vi "Common_UpdateAttributes.vi"(1 "ClassPath/LvClassRef":variant, 2 "NewAttributes":string, 3 "ClassInfo":T4[](array[typedef]), 5 "error in (no error)":errorcluster, 6 "Don't Prompt (False)":bool, 7 "Attributes":T1[](array[typedef]), 8 "Stereotype":string, 9 "Ctl-Description":string) -> (15 "CtlPath":path, 18 "Cancel":bool, 19 "error out":errorcluster)   [LabVIEW 2020] (continued)
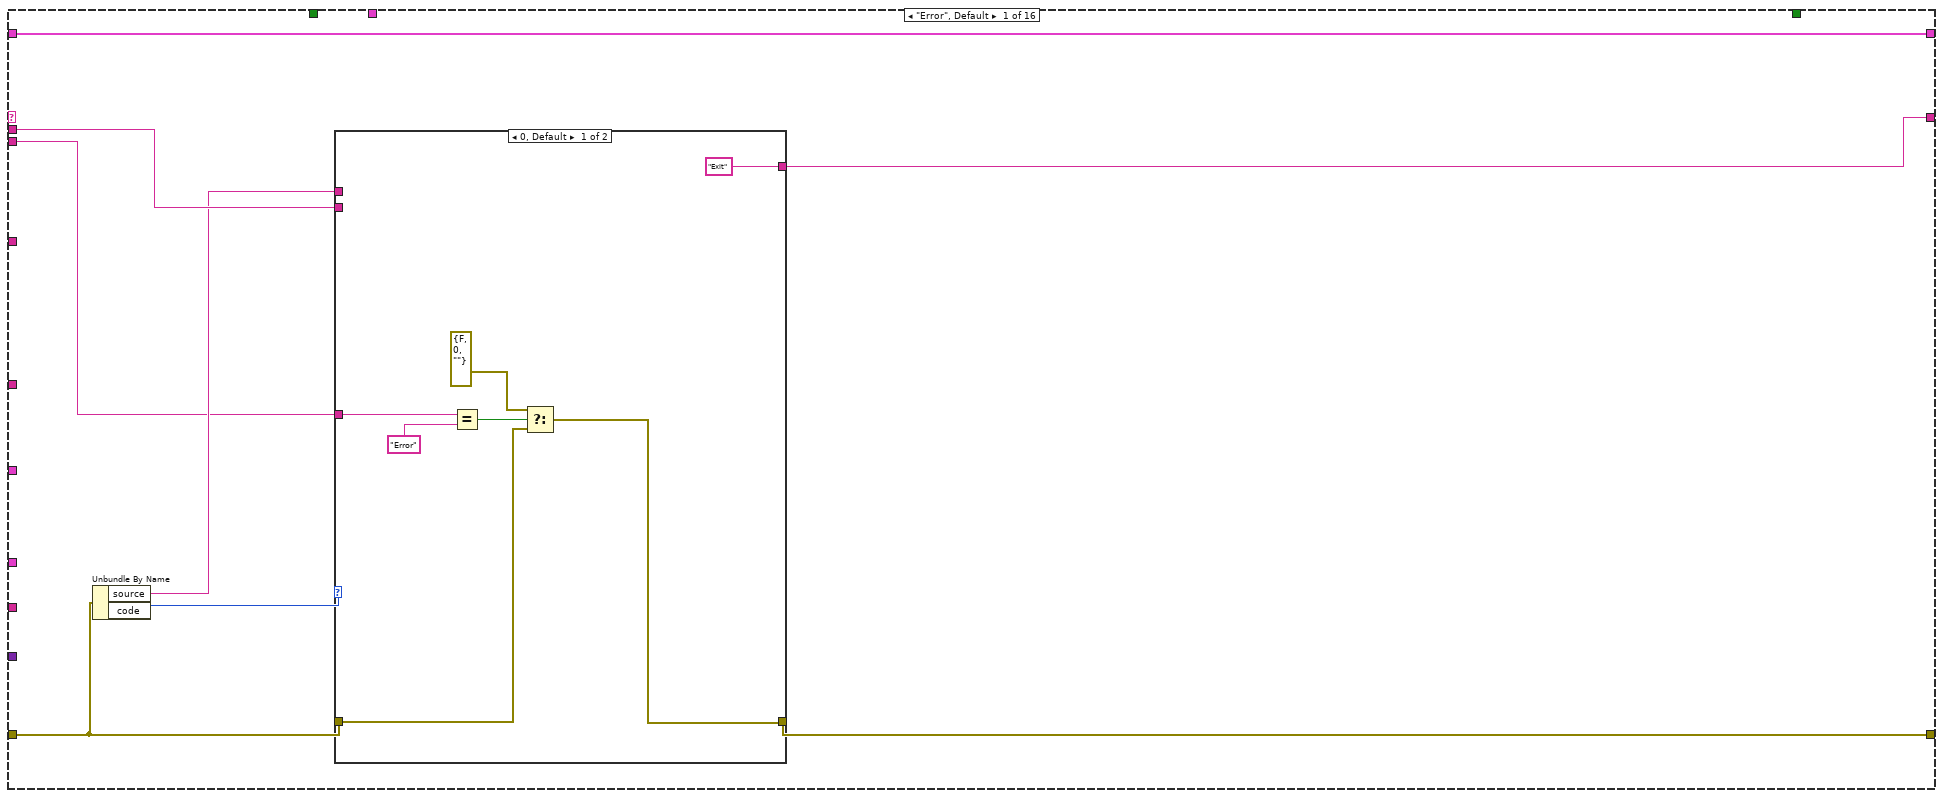
[diagram p3: hidden frame]
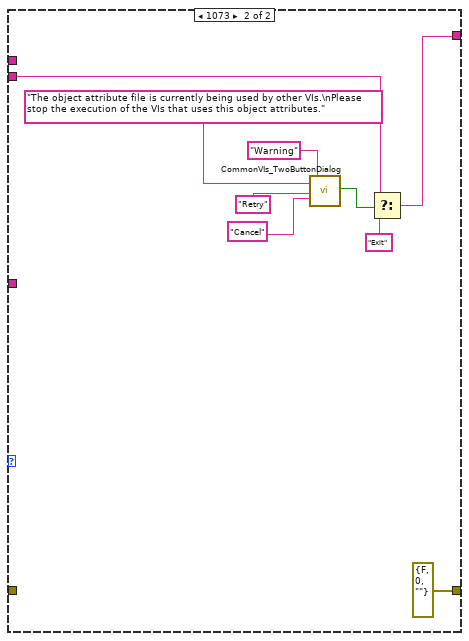
[diagram p4: hidden frame]
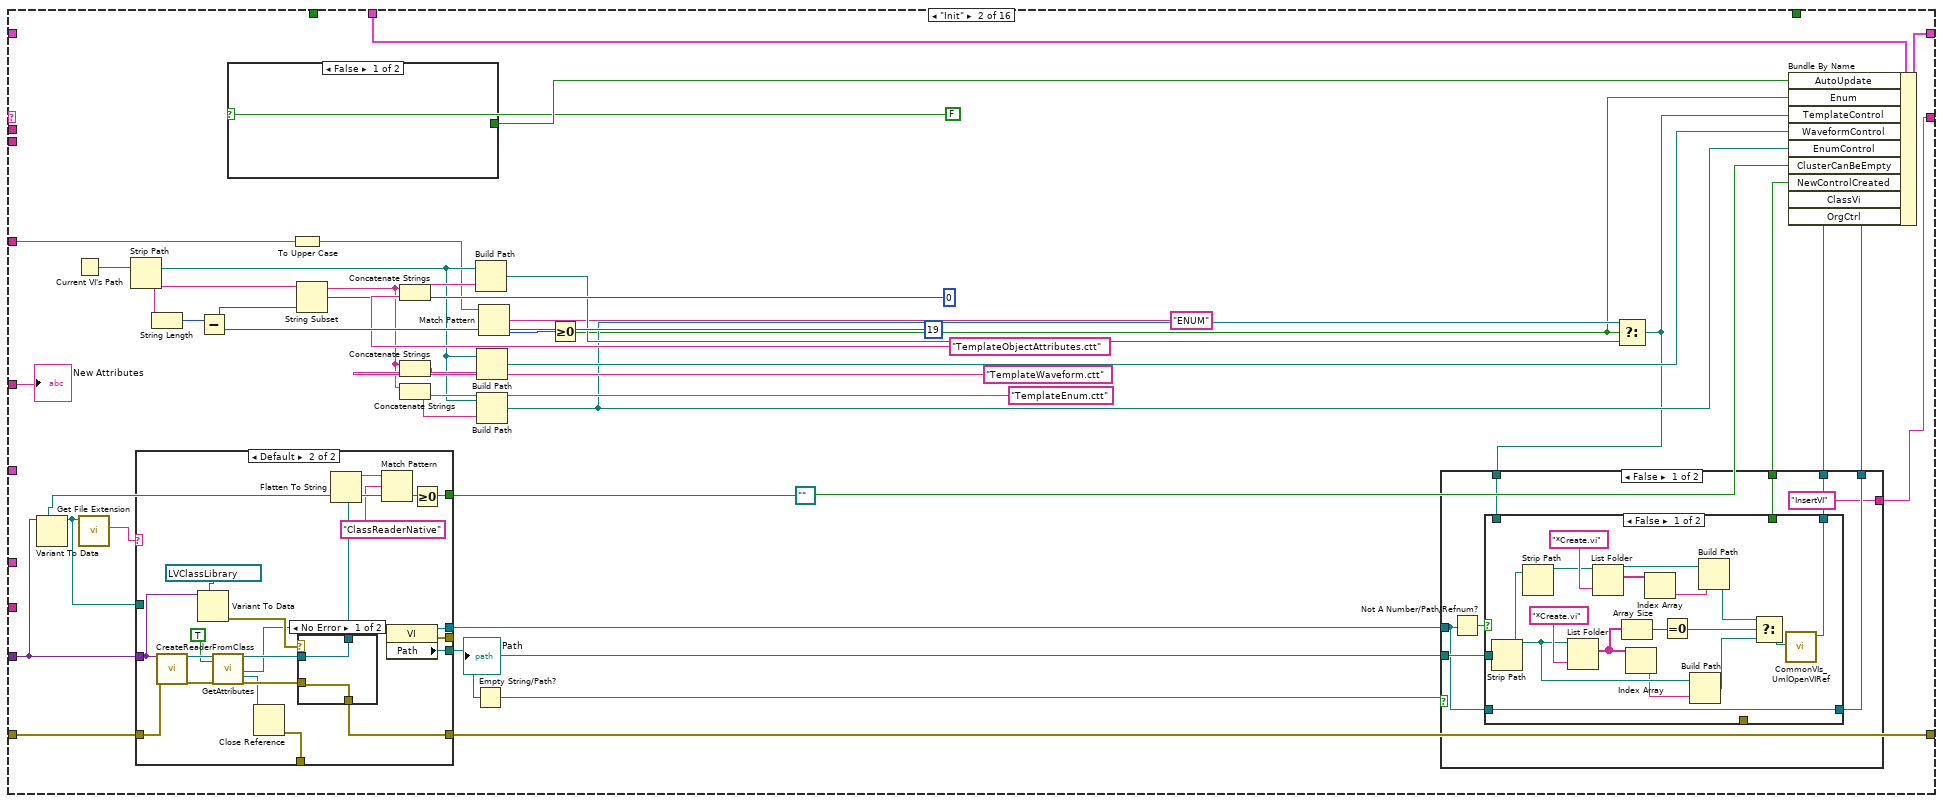
[diagram p5: hidden frame]
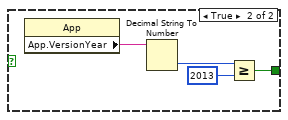
[diagram p6: hidden frame]
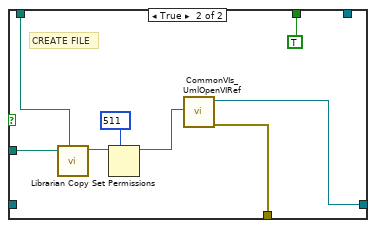
[diagram p7: hidden frame]
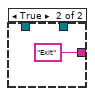
[diagram p8: hidden frame]
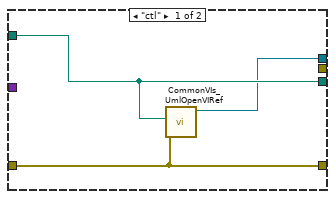
[diagram p9: hidden frame]
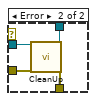
[diagram p10: hidden frame]
                  n285 = Close Reference(reference=w814, error in (no error)=w826) -> (error out=w832:errorcluster)
                  n286 = for {
                    tunnel: w806 -> [w838] mode=indexing
                    tunnel: w799 -> [_]
                    n287 = Close Reference(reference=w838) -> ()  [unwired: 1 in, 1 out]
                  }
                  n288 = invoke on="EmptyClip" class="App" method="Clipboard.Empty"(error in=w832) -> (error out=w833:errorcluster)  [unwired: 2 in, 2 out]
                }
              }
              n289 = property class="Ctl"(reference=w535, error in=w544, "Label.Text"=w515, "Auto-Update From Typedef"=TRUE ("Label.Visible")) -> (reference out=w540:refnum<vi>, error out=w545:errorcluster)
              n290 = property class="Ctl"(reference=w540, error in=w545, "Label.Text"=w515, "Label.Visible"=TRUE) -> (reference out=w541:refnum<vi>, error out=w543:errorcluster)
            }
            n291 = Array Size(array=w487) -> (size(s)=w484:i32)
            n292 = Equal?(x=w485, y=w484) -> (x = y?=w483:bool)
            n293 = And Array Elements(Boolean array=w487) -> (logical AND=w488:bool)
            n294 = And(x=w483, y=w488) -> (x .and. y?=w482:bool)
            n295 = Build Array (concatenate)(w502, w500) -> (w501:refnum<vi>[])
            n296 = Bundle By Name(cluster=w491, "NoUpdate"=w482, "AddedCtrls"=w501) -> (w503:T5)
          }
          frame "Move Controls" {
            n297 = Unbundle By Name(w845) -> ("NewCtrl"=w856:refnum<vi>, "NewCluster"=w855:refnum<vi>, "OrgCtrl"=w852:refnum<vi>, "OrgCluster"=w853:refnum<vi>, "NewEnum"=w846:refnum<vi>)
            n298 = property class="VI"(reference=w852) -> ("Front Panel Window:Origin"=w854:T13)  [unwired: 1 in, 2 out]
            n299 = property class="VI"(reference=w856) -> ("Front Panel Window:Origin"=w847:T13)  [unwired: 1 in, 2 out]
            n300 = property class="Clust"(reference=w853, "Position"=w854) -> ()  [unwired: 1 in, 2 out]
            n301 = property class="Clust"(reference=w855, "Position"=w847) -> ()  [unwired: 1 in, 2 out]
            n302 = property class="Enum"(reference=w846, "Position"=w847) -> ()  [unwired: 1 in, 2 out]
            n303 = case shown="True" FALSE {
              tunnel: [_ w858] -> w841
              frame False {
              }
              frame True {
                n304 = property class="App"() -> ("App.VersionYear"=w861:string)  [unwired: 2 in, 2 out]
                n305 = Decimal String To Number(string=w861) -> (number=w860:i32)  [unwired: 2 in, 1 out]
                n306 = Greater Or Equal?(x=w860, y=2013) -> (x >= y?=w858:bool)
              }
            }
            n307 = Unbundle By Name(w845) -> ("NoUpdate"=w843:bool, "AutoUpdate"=w842:bool, "NewControlCreated"=w839:bool)
            n308 = Compound Arithmetic op=OR(w848, w843, w842, w839, w841) -> (w844:bool)
            n309 = Select(t="SaveCtrl" ("y"), s=w844, f="Idle" ("y")) -> (s? t:f=w849:string)
          }
          frame "Idle" {
            n310 = Unbundle By Name(w870) -> ("NewCluster"=w869:refnum<vi>, "OrgCtrl"=w862:refnum<vi>)  [unwired: 1 out]
            n311 = while {
              tunnel: [w881] -> w871
              tunnel: w862 -> [w880]
              stop <- w879 stop-if-true
              n312 = event shown="[3] Panel Close?" {
                selector: _ -> [_ _ _ _]
                dyn-events: _ -> [_ _ _ _]
                timeout: 500 -> [_ _ _ _]
                tunnel: ["Cancel" _ _ TRUE ("Cancel")] -> w881
                tunnel: w880 -> [_ w895 _ _]
                tunnel: [TRUE _ _ TRUE] -> w879
                event "OK", "Cancel": Value Change {
                  n313 = event-data() -> ()  [unwired: 2 out]
                  n314 = case shown="True" "OK" {
                    frame False {
                    }
                    frame True {
                      n315 = call <vilib>:"Set Busy.vi"() -> ()  [unwired: 4 in, 8 out]
                    }
                  }
                }
                event "Backup": Value Change {
                  n316 = event-data() -> ()  [unwired: 2 out]
                  n317 = call <vilib>:"Dflt Data Dir.vi"() -> ("App:Default Data Directory"=w905:path)
                  n318 = Format Date/Time String(time format string (%c)="%y%m%d_%H%M%S_") -> (date/time string=w900:string)  [unwired: 2 out]
                  n319 = property class="VI"(reference=w895) -> (reference out=w896:refnum<vi>, error out=w906:errorcluster, "VI Name"=w887:string)  [unwired: 1 in]
                  n320 = Build Path(base path=w905, name or relative path="Backup") -> (appended path=w901:path)
                  n321 = Match Pattern(string=w887, regular expression=":") -> (after substring=w886:string)  [unwired: 4 out]
                  n322 = Create Folder(path (use dialog)=w901) -> (created path=w890:path)  [unwired: 1 in, 3 out]
                  n323 = Concatenate Strings(w900, w886) -> (w891:string)
                  n324 = Build Path(base path=w890, name or relative path=w891) -> (appended path=w893:path)
                  n325 = Format Into String(format string="Do you want to save a backup file\nof the original control here.\n\n%s", w893) -> (resulting string=w902:string)  [unwired: 2 in, 1 out]
                  n326 = Two Button Dialog(message=w902, 1:"No" ("F button name (\"Cancel\")"), 2:"Yes" ("T button name (\"OK\")")) -> (T button?=w894:bool)
                  n327 = case shown="False" w894 {
                    tunnel: w893 -> [_ w914]
                    tunnel: [w910 w914] -> w892
                    tunnel: w891 -> [w912 _]
                    tunnel: w890 -> [w911 _]
                    tunnel: [w909 _] -> w889
                    tunnel: "Select backup file path" ("prompt") -> [w908 _]
                    frame False {
                      (unwired) T14."new or existing file" ("select mode (2)")
                      n328 = File Dialog(5:"Save" ("button label"), 6:"*.ctl" ("default name"), 7:w908, 9:w912, 11:w911) -> (1:w909:bool, 3:w910:path)  [unwired: 1 in, 3 out]
                    }
                    frame True {
                    }
                  }
                  n329 = case shown="False" w889 {
                    tunnel: w906 -> [w920 w922]
                    tunnel: w896 -> [w916 w921]
                    tunnel: w892 -> [w918 _]
                    tunnel: [w917 w921] -> _
                    tunnel: [w919 w922] -> _
                    frame False {
                      n330 = invoke class="VI" method="Save.Instrument"(reference=w916, error in=w920, "Path to saved file"=w918, "Save a Copy"=TRUE) -> (reference out=w917:refnum<vi>, error out=w919:errorcluster)  [unwired: 2 in, 4 out]
                    }
                    frame True {
                    }
                  }
                }
                event Timeout {
                  n331 = event-data() -> ()  [unwired: 2 out]
                  n332 = property class="VI"("Front Panel Window:Is Frontmost"=TRUE) -> ()  [unwired: 2 in, 2 out]
                }
                event Panel Close? {
                  n333 = event-data() -> ()  [unwired: 2 out]
                  n334 = event-data("Discard?"=TRUE) -> ()  [unwired: 1 in, 1 out]
                }
              }
            }
            n335 = property class="Clust"(reference=w869, "Auto Sizing"=u32 3) -> ("Controls[]"=w863:refnum<vi>[])  [unwired: 1 in, 2 out]
            n336 = Index Array(array=w863) -> (element=w867:refnum<vi>)  [unwired: 1 in]
            n337 = property class="Ctl"(reference=w867) -> (reference out=w866:refnum<vi>, "Position:Left"=w865:i32)  [unwired: 1 in, 1 out]
            n338 = Increment(x=w865) -> (x+1=w864:i32)
            n339 = property class="Ctl"(reference=w866, "Position:Left"=w864) -> (error out=w876:errorcluster)  [unwired: 1 in, 1 out]
            n340 = for {
              tunnel: w863 -> [w927] mode=indexing
              tunnel: w876 -> [_]
              n341 = Close Reference(reference=w927) -> ()  [unwired: 1 in, 1 out]
            }
            n342 = invoke class="VI" method="FP.Open"() -> ()  [unwired: 5 in, 5 out]
            n343 = Bundle By Name(cluster=w870, "Cancel"=w871) -> (w872:T5)
            n344 = Select(t="Exit" ("y"), s=w871, f="SaveCtrl" ("y")) -> (s? t:f=w873:string)
          }
          frame "SaveCtrl" {
            n345 = Unbundle By Name(w935) -> ("NewEnum"=w929:refnum<vi>, "OrgCluster"=w933:refnum<vi>, "OrgCtrl"=w928:refnum<vi>)  [unwired: 1 out]
            n346 = stacked-sequence {
              tunnel: w940 -> [w945]
              tunnel: [w945] -> w936
              tunnel: [w944] -> _
              tunnel: [w943] -> _
              frame #0 {
                n347 = invoke on="Attribute Before" class="SubPanel" method="Remove VI"() -> (error out=w944:errorcluster)  [unwired: 3 in, 2 out]
                n348 = invoke on="Attribute After" class="SubPnl" method="Remove VI"() -> (error out=w943:errorcluster)  [unwired: 3 in, 2 out]
              }
            }
            n349 = property class="VI"(reference=w928, error in=w936, "Front Panel Window:Origin"=cluster{"Horizontal":i16, "Vertical":i16} {"Horizontal"=0, "Vertical"=0}) -> (error out=w937:errorcluster)  [unwired: 1 out]
            n350 = property class="Clust"(reference=w933, error in=w937, "Position"=cluster{"Left":i32, "Top":i32} {"Left"=5, "Top"=5}) -> (error out=w938:errorcluster)  [unwired: 1 out]
            n351 = property class="Enum"(reference=w929, error in=w937, "Position"=cluster{"Left":i32, "Top":i32} {"Left"=5, "Top"=5}) -> (error out=w939:errorcluster)  [unwired: 1 out]
            n352 = stacked-sequence {
              tunnel: w937 -> [w941]
              tunnel: w939 -> [_]
              tunnel: w938 -> [_]
              frame #0 {
                n353 = disable-structure shown="Disabled" {
                  disable-tunnel: w941 -> [w942 _]
                  frame Disabled {
                    n354 = invoke class="VI" method="Save.Instrument"(error in=w942) -> ()  [unwired: 5 in, 6 out]
                  }
                  frame Enabled {
                  }
                }
              }
            }
          }
          frame "ReplaceCtrl" {
            n355 = Unbundle By Name(w981) -> ("Enum"=w969:bool, "OrgEnum"=w966:refnum<vi>, "OrgCtrl"=w957:refnum<vi>, "OrgCluster"=w965:refnum<vi>, "NewCtrl"=w958:refnum<vi>, "NewCluster"=w972:refnum<vi>, "NewEnum"=w970:refnum<vi>, "ClassVi"=w977:refnum<vi>, "NewControlCreated"=w946:bool)
            n356 = property class="Clust"(reference=w965) -> (reference out=w964:refnum<vi>, "Label.Text"=w963:string)  [unwired: 1 in, 1 out]
            n357 = property class="VI"(reference=w958, error in=w1014) -> (reference out=w979:refnum<vi>, error out=w1001:errorcluster, "Front Panel"=w971:refnum<vi>)
            n358 = invoke class="Enum" method="Delete"(reference=w966, error in=w1001) -> (reference out=w968:refnum<vi>, error out=w1002:errorcluster)  [unwired: 1 in, 1 out]
            n359 = invoke class="Clust" method="Delete"(reference=w964, error in=w1001) -> (reference out=w967:refnum<vi>, error out=w1003:errorcluster)  [unwired: 1 in, 1 out]
            n360 = Close Reference(reference=w967, error in (no error)=w1003) -> (error out=w999:errorcluster)
            n361 = Close Reference(reference=w968, error in (no error)=w1002) -> (error out=w998:errorcluster)
            n362 = case shown="Error" w1002 {
              selector: w1002 -> [w1032 _]
              tunnel: w1003 -> [_ w1033]
              tunnel: [w1032 w1033] -> w1004
              tunnel: w999 -> [_ _]
              tunnel: w998 -> [_ _]
              frame No Error {
              }
              frame Error {
              }
            }
            n363 = case shown="False" w969 {
              tunnel: w972 -> [_ w1051]
              tunnel: [w1050 w1054] -> w1005
              tunnel: w970 -> [w1047 _]
              tunnel: w1004 -> [w1049 w1053]
              frame True {
                n364 = property class="Enum"(reference=w1047, error in=w1049, "Selected"=TRUE) -> (error out=w1050:errorcluster)  [unwired: 1 out]
              }
              frame False {
                n365 = property class="Clust"(reference=w1051, error in=w1053, "Selected"=TRUE) -> (error out=w1054:errorcluster)  [unwired: 1 out]
              }
            }
            n366 = invoke class="Pnl" method="Copy Selection"(reference=w971, error in=w1005) -> (reference out=w982:refnum<vi>, error out=w1013:errorcluster)  [unwired: 1 in, 1 out]
            n367 = Close Reference(reference=w982, error in (no error)=w1013) -> (error out=w996:errorcluster)
            n368 = invoke class="VI" method="FP.Open"(reference=w957, error in=w996, "State"=T8."Hidden") -> (reference out=w956:refnum<vi>, error out=w997:errorcluster)  [unwired: 2 in, 3 out]
            n369 = property class="VI"(reference=w956, error in=w997) -> (error out=w1016:errorcluster, "Front Panel"=w985:refnum<vi>)  [unwired: 1 out]
            n370 = invoke class="Pnl" method="Paste Selection"(reference=w985, error in=w1016, "Pos"=cluster{"Left":i32, "Top":i32} {"Left"=20, "Top"=40}) -> (reference out=w983:refnum<vi>, error out=w1015:errorcluster)  [unwired: 2 in, 3 out]
            n371 = Close Reference(reference=w983, error in (no error)=w1015) -> (error out=w1012:errorcluster)
            n372 = invoke class="App" method="Clipboard.Empty"(error in=w1012) -> (error out=w1007:errorcluster)  [unwired: 2 in, 2 out]
            n373 = property class="VI"(reference=w957, error in=w1007) -> (reference out=w947:refnum<vi>, error out=w1010:errorcluster, "Front Panel"=w975:refnum<vi>)
            n374 = case shown="\"\"" w950 {
              selector: w950 -> [_ w1022]
              tunnel: w947 -> [w1021 w1024]
              tunnel: [w1021 w1023] -> w951
              frame "" {
              }
              frame Default {
                n375 = property class="VI"(reference=w1024, "Description"=w1022) -> (reference out=w1023:refnum<vi>)  [unwired: 1 in, 1 out]
              }
            }
            n376 = property class="Pnl"(reference=w975, error in=w1010) -> (reference out=w973:refnum<vi>, error out=w1009:errorcluster, "Controls[]"=w974:refnum<vi>[])
            n377 = Index Array(array=w974) -> (element=w976:refnum<vi>)  [unwired: 1 in]
            n378 = case shown="False" w969 {
              tunnel: w1009 -> [w1042 w1046]
              tunnel: w976 -> [w1040 _]
              tunnel: w963 -> [w1034 _]
              tunnel: [w1042 w1046] -> w986
              frame False {
                w1041 = refnum<vi> refnum  # Cluster
                n379 = To More Specific Class(target class=w1041, reference=w1040, error in=w1042) -> (specific class reference=w1039:refnum<vi>, error out=w1044:errorcluster)
                n380 = property class="Clust"(reference=w1039, error in=w1044, "Auto Sizing"=u32 0) -> (reference out=w1037:refnum<vi>, error out=w1045:errorcluster)
                n381 = property class="Clust"(reference=w1037, error in=w1045, "Auto Sizing"=u32 3) -> (reference out=w1035:refnum<vi>, error out=w1043:errorcluster)
                n382 = property class="Clust"(reference=w1035, error in=w1043, "Label.Text"=w1034) -> ()  [unwired: 2 out]
              }
              frame True {
              }
            }
            n383 = case shown="False" w946 {
              tunnel: w947 -> [_ w1018]
              tunnel: [w1017 w1020] -> w987
              tunnel: w986 -> [w1017 w1020]
              frame False {
              }
              frame True {
                n384 = call <resource>:"GDSIconEditor_CreateVIIcon.vi"("ViRef(IgnoreIfNotWired)"=w1018, "AutomaticUpdateNoQuestionsAsked(False)"=TRUE) -> ()  [unwired: 9 in, 1 out]
              }
            }
            n385 = Select(t=w1007, s=w987, f=w987) -> (s? t:f=w1006:errorcluster)
            n386 = invoke class="VI" method="Save.Instrument"(reference=w951, error in=w1006) -> (reference out=w959:refnum<vi>, error out=w990:errorcluster)  [unwired: 4 in, 4 out]
            n387 = property class="VI"(reference=w959, error in=w990) -> (error out=w991:errorcluster, "Library"=w962:refnum<vi>, "Path"=w948:path)  [unwired: 1 out]
            n388 = To More Specific Class(target class=refnum<vi> refnum ("ClassRefIn"), reference=w962, error in=w991) -> (specific class reference=w960:refnum<vi>, error out=w1000:errorcluster)
            n389 = case shown="Error" w1000 {
              selector: w1000 -> [w1029 _]
              tunnel: w960 -> [w1026 w1030]
              tunnel: w991 -> [_ w1031]
              tunnel: [w1027 w1031] -> w989
              frame No Error {
                n390 = call <resource>:"GDSLvClass_SaveEverythingInClass.vi"("ClassRefIn"=w1026, "error in"=w1029) -> ("ClassRefOut"=w1025:refnum<vi>, "error out"=w1028:errorcluster)  [unwired: 1 in, 15 out]
                n391 = Close Reference(reference=w1025, error in (no error)=w1028) -> (error out=w1027:errorcluster)
              }
              frame Error {
                n392 = Close Reference(reference=w1030) -> ()  [unwired: 1 in, 1 out]
              }
            }
            n393 = Close Reference(reference=w974, error in (no error)=w989) -> (error out=w1008:errorcluster)
            n394 = Close Reference(reference=w973, error in (no error)=w1008) -> (error out=w988:errorcluster)
            n395 = Bundle By Name(cluster=w981, "CtlPath"=w948) -> (w949:T5)
            n396 = Close Reference(reference=w979, error in (no error)=w988) -> (error out=w994:errorcluster)
            n397 = invoke class="VI" method="Save.Instrument"(reference=w977, error in=w994) -> (reference out=w978:refnum<vi>, error out=w1011:errorcluster)  [unwired: 4 in, 4 out]
            n398 = Close Reference(reference=w978, error in (no error)=w1011) -> ()  [unwired: 1 out]
            n399 = invoke class="VI" method="CtlVIApplyChanges"(reference=w947, error in=w994) -> (reference out=w953:refnum<vi>, error out=w993:errorcluster)  [unwired: 1 in, 1 out]
            n400 = call <resource>:"CommonVIs_Wait.vi"("error in"=w993) -> ("error out"=w992:errorcluster)  [unwired: 9 in]
            n401 = invoke class="VI" method="Save.Instrument"(reference=w953, error in=w992) -> (reference out=w952:refnum<vi>)  [unwired: 4 in, 5 out]
            n402 = invoke class="VI" method="FP.Close"(reference=w952) -> (reference out=w955:refnum<vi>, error out=w995:errorcluster)  [unwired: 2 in, 1 out]
            n403 = Close Reference(reference=w955, error in (no error)=w995) -> ()  [unwired: 1 out]
          }
          frame "AddToProject?" {
            n404 = Unbundle By Name(w1056) -> ("NewControlCreated"=w1055:bool)
            n405 = case shown="True" w1055 {
              tunnel: w1059 -> [w1060 w1066]
              tunnel: [w1060 w1064] -> w1058
              frame False {
              }
              frame True {
                n406 = call <resource>:"CommonVIs_UmlOpenVIRef.vi"("error in"=w1066) -> ("error out"=w1067:errorcluster, "ProjectNameOut"=w1063:string)  [unwired: 3 in, 6 out]
                n407 = call <resource>:"GDSProject_GetProjects.vi"("GetProjectRefByName"=w1063, "error in (no error)"=w1067) -> ("Project Refnum"=w1062:refnum<vi>, "error out"=w1065:errorcluster)  [unwired: 1 in, 15 out]
                n408 = Not A Number/Path/Refnum?(number/path/refnum=w1062) -> (NaN/Path/Refnum?=w1061:bool)
                n409 = case shown="False" w1061 {
                  tunnel: w1062 -> [w1087 _]
                  tunnel: w1065 -> [w1097 w1116]
                  tunnel: [w1090 w1116] -> w1064
                  tunnel: [w1091 _] -> _
                  frame False {
                    w1075 = refnum<vi> refnum  # LVClassLibrary
                    n410 = property class="Project"(reference=w1087, error in=w1097) -> (reference out=w1073:refnum<vi>, error out=w1096:errorcluster, "My Computer"=w1085:refnum<vi>)
                    n411 = local read "Path"() -> (w1078:path)
                    n412 = invoke class="TargetItem" method="Get All Descendents"(reference=w1085, error in=w1096, "Type"="lvclass") -> (reference out=w1077:refnum<vi>, error out=w1088:errorcluster, "All Descendents"=w1084:refnum<vi>[])  [unwired: 4 in, 4 out]
                    n413 = Strip Path(path=w1078) -> (stripped path=w1083:path)  [unwired: 1 out]
                    n414 = for {
                      tunnel: w1084 -> [w1115] mode=indexing
                      tunnel: w1083 -> [w1112]
                      tunnel: [w1111] -> w1082 mode=indexing
                      tunnel: [w1110] -> w1068 mode=indexing
                      n415 = property class="ProjectItem"(reference=w1115) -> (reference out=w1110:refnum<vi>, "Path"=w1114:path)  [unwired: 1 in, 1 out]
                      n416 = Strip Path(path=w1114) -> (stripped path=w1113:path)  [unwired: 1 out]
                      n417 = call <vilib>:"Compare Two Paths.vi"("Path 2"=w1112, "Path 1"=w1113) -> ("Path 2 Relative to Path 1?"=w1111:bool)  [unwired: 1 in, 8 out]
                    }
                    n418 = Search 1D Array(1D array=w1082, element=TRUE) -> (index of element=w1080:i32)  [unwired: 1 out]
                    n419 = case shown="0, Default" w1080 {
                      selector: w1080 -> [w1107 _]
                      tunnel: w1068 -> [w1108 _]
                      tunnel: [w1106 w1109] -> w1079
                      tunnel: w1077 -> [_ w1109]
                      frame 0, Default {
                        n420 = Index Array(array=w1108, index=w1107) -> (element=w1106:refnum<vi>)
                      }
                      frame -1 {
                      }
                    }
                    n421 = invoke class="ProjectItem" method="AddFile"(reference=w1079, error in=w1088, "Path"=w1078) -> (reference out=w1076:refnum<vi>, error out=w1089:errorcluster, "AddFile"=w1072:refnum<vi>)  [unwired: 1 in, 1 out]
                    n422 = property class="ProjectItem"(reference=w1072) -> (reference out=w1069:refnum<vi>, "Reference"=w1071:refnum<vi>)  [unwired: 1 in, 1 out]
                    n423 = To More Specific Class(target class=w1075, reference=w1076, error in=w1089) -> (specific class reference=w1074:refnum<vi>, error out=w1095:errorcluster)
                    n424 = invoke class="VI" method="Save.Instrument"(reference=w1071) -> (reference out=w1070:refnum<vi>, error out=w1093:errorcluster)  [unwired: 5 in, 4 out]
                    n425 = case shown="Error" w1095 {
                      tunnel: w1074 -> [w1103 _]
                      tunnel: [w1104 w1105] -> w1094
                      tunnel: w1088 -> [_ w1105]
                      frame No Error {
                        n426 = invoke class="LVClassLibrary" method="Save"(reference=w1103) -> (error out=w1104:errorcluster)  [unwired: 3 in, 3 out]
                      }
                      frame Error {
                      }
                    }
                    n427 = Close Reference(reference=w1070, error in (no error)=w1093) -> (error out=w1092:errorcluster)
                    n428 = stacked-sequence {
                      tunnel: w1077 -> [w1100]
                      tunnel: [w1101] -> w1090
                      tunnel: w1073 -> [w1098]
                      tunnel: w1094 -> [w1101]
                      frame #0 {
                        n429 = invoke class="Project" method="Save"(reference=w1098) -> (reference out=w1099:refnum<vi>, error out=w1102:errorcluster)  [unwired: 3 in, 2 out]
                        n430 = Close Reference(reference=w1100) -> ()  [unwired: 1 in, 1 out]
                        n431 = Close Reference(reference=w1099, error in (no error)=w1102) -> ()  [unwired: 1 out]
                      }
                    }
                    n432 = Close Reference(reference=w1068, error in (no error)=w1090) -> ()  [unwired: 1 out]
                    n433 = Close Reference(reference=w1069, error in (no error)=w1092) -> (error out=w1091:errorcluster)
                  }
                  frame True {
                  }
                }
              }
            }
          }
        }
        n434 = Select(t="Error", s=w63, f=w56) -> (s? t:f=w57:string)
        n435 = Equal?(x=w56, y="Exit") -> (x = y?=w54:bool)
      }
    }
    frame Error {
    }
  }
  "error out" <- w31
  n436 = Unbundle By Name(w22) -> ("CtlPath"=→"CtlPath":path, "ClassVi"=w7:refnum<vi>, "NewCtrl"=w8:refnum<vi>, "NewCluster"=w9:refnum<vi>, "NewEnum"=w10:refnum<vi>, "OrgEnum"=w11:refnum<vi>, "AddedCtrls"=w6:refnum<vi>[], "OrgCtrl"=w21:refnum<vi>, "OrgCluster"=w18:refnum<vi>, "Cancel"=w15:bool, "NewControlCreated"=w14:bool)
  n437 = And(x=w15, y=w14) -> (x .and. y?=w13:bool)
  n438 = case shown="True" w13 {
    tunnel: [_ w1119] -> _
    frame False {
    }
    frame True {
      n439 = local read "Path"() -> (w1118:path)
      n440 = Delete(path (use dialog)=w1118) -> (error out=w1119:errorcluster)  [unwired: 1 in, 5 out]
    }
  }
  n441 = Close Reference(reference=w8) -> (error out=w26:errorcluster)  [unwired: 1 in]
  n442 = Close Reference(reference=w9) -> (error out=w27:errorcluster)  [unwired: 1 in]
  n443 = Close Reference(reference=w7) -> (error out=w25:errorcluster)  [unwired: 1 in]
  n444 = Close Reference(reference=w10) -> (error out=w28:errorcluster)  [unwired: 1 in]
  n445 = Close Reference(reference=w11) -> ()  [unwired: 1 in, 1 out]
  n446 = Close Reference(reference=w18) -> (error out=w30:errorcluster)  [unwired: 1 in]
  n447 = Close Reference(reference=w21) -> (error out=w29:errorcluster)  [unwired: 1 in]
  n448 = stacked-sequence {
    tunnel: w30 -> [w1121]
    tunnel: w29 -> [_]
    tunnel: w28 -> [_]
    tunnel: w27 -> [_]
    tunnel: w26 -> [_]
    tunnel: w25 -> [_]
    tunnel: w6 -> [w1120]
    tunnel: [w1121] -> w24
    frame #0 {
      n449 = Close Reference(reference=w1120) -> ()  [unwired: 1 in, 1 out]
    }
  }
  n450 = stacked-sequence {
    tunnel: w15 -> [w1123]
    tunnel: [FALSE ("Front Panel Window:Open")] -> w12
    tunnel: w24 -> [_]
    tunnel: [w1125] -> _
    tunnel: [w1124] -> _
    frame #0 {
      n451 = call <vilib>:"Unset Busy.vi"() -> ()  [unwired: 2 in, 10 out]
      n452 = invoke on="Attribute Before" class="SubPanel" method="Remove VI"() -> (error out=w1125:errorcluster)  [unwired: 3 in, 2 out]
      n453 = invoke on="Attribute After" class="SubPnl" method="Remove VI"() -> (error out=w1124:errorcluster)  [unwired: 3 in, 2 out]
      "Cancel" <- w1123
    }
  }
  n454 = property class="VI"("Front Panel Window:Open"=w12) -> ()  [unwired: 2 in, 2 out]
